vi "PCO_SetConfig.vi"(8 "error in":errorcluster caption="entrée d'erreur", 11 "PCO_Config":T3 {"TriggerMode" items=["auto sequence", "software trigger", "external exposure start", "external exposure control"]}) -> (0 "error out":errorcluster caption="sortie d'erreur", 1 "PCO_Config 2":T3 {"TriggerMode" items=["auto sequence", "software trigger", "external exposure start", "external exposure control"]}, 2 "Trigger externe?":bool, 3 "configuration":T2={"exposure_time_s"=nan, "delay_time_s"=nan, "roi"={"x0"=18446744073709551615, "y0"=18446744073709551615, "x1"=18446744073709551615, "y1"=18446744073709551615}, "timestamp_mode"=65535, "pixelrate"=4294967295, "conversion_factor"=0.7, "trigger_mode"=65535, "acquire_mode"=65535, "acquire_sequence_number"=1, "metadata_mode"=65535, "noisefilter_mode"=65535, "pixel_format"=0, "binning"={"vert"=0, "horz"=0, "mode"=0}, "auto_exposure"={"region"=0, "min_exposure_s"=0.001, "max_exposure_s"=0.1}} {"conversion_factor" format="%.2g"; "auto_exposure"."region" items=["balanced", "center_based", "corner_based", "full", "custom"]; "binning"."mode" items=["sum", "average"]; "noisefilter_mode" items=["Undefined"=65535, "OFF"=0, "ON"=1]; "exposure_time_s" format="%#_6f"; "timestamp_mode" items=["Undefined"=65535, "OFF"=0, "Binary"=1, "Binary+ASCII"=2, "ASCII"=3]; "acquire_mode" items=["Undefined"=65535, "auto"=0, "external"=1, "external modulate"=2]; "trigger_mode" items=["Undefined"=65535, "auto sequence"=0, "software trigger"=1, "external exposure start & software trigger"=2, "external exposure control"=3, "external synchronized"=4, "fast external exposure control"=5, "external CDS control"=6, "slow external exposure control"=7, "external synchronized HDSDI"=258]; "metadata_mode" items=["Undefined"=65535, "OFF"=0, "ON"=1]})   [LabVIEW 2026]
uses:
  Controls/PCO_Config.ctl
  pco.labview/camera/Controls/binning.ctl
  pco.labview/camera/Camera.lvclass
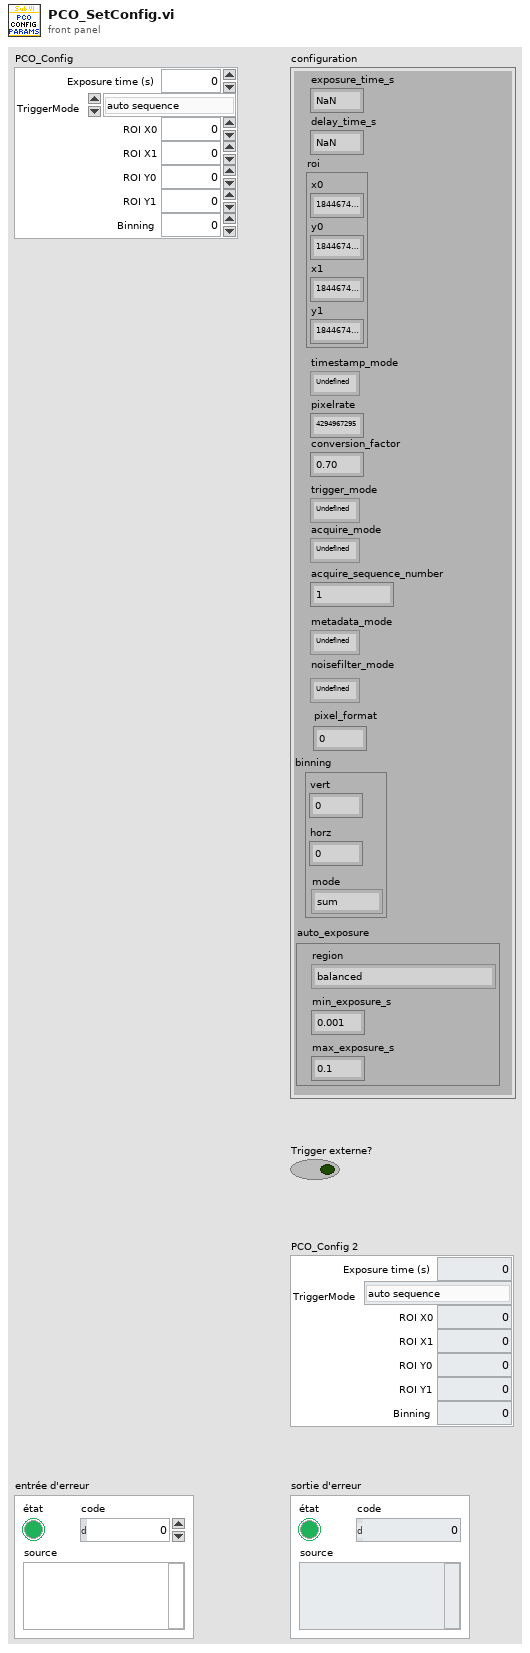
[diagram p1: front panel]
types:
  T1 = typedef "Camera.lvclass/binning.ctl" = cluster{"vert":u16, "horz":u16, "mode":u16}
  T2 = cluster{"exposure_time_s":dbl, "delay_time_s":dbl, "roi":cluster{"x0":u64, "y0":u64, "x1":u64, "y1":u64}, "timestamp_mode":u16, "pixelrate":u32, "conversion_factor":sgl, "trigger_mode":u16, "acquire_mode":u16, "acquire_sequence_number":u32, "metadata_mode":u16, "noisefilter_mode":u16, "pixel_format":u32, "binning":T1, "auto_exposure":cluster{"region":u16, "min_exposure_s":dbl, "max_exposure_s":dbl}}
  T3 = typedef "PCO_Config.ctl" = cluster{"Exposure time (s)":dbl, "TriggerMode":u16, "ROI X0":u16, "ROI Y0":u16, "ROI X1":u16, "ROI Y1":u16, "Binning":u8}
  T4 = enum16{"auto sequence", "software trigger", "external exposure start", "external exposure control"}
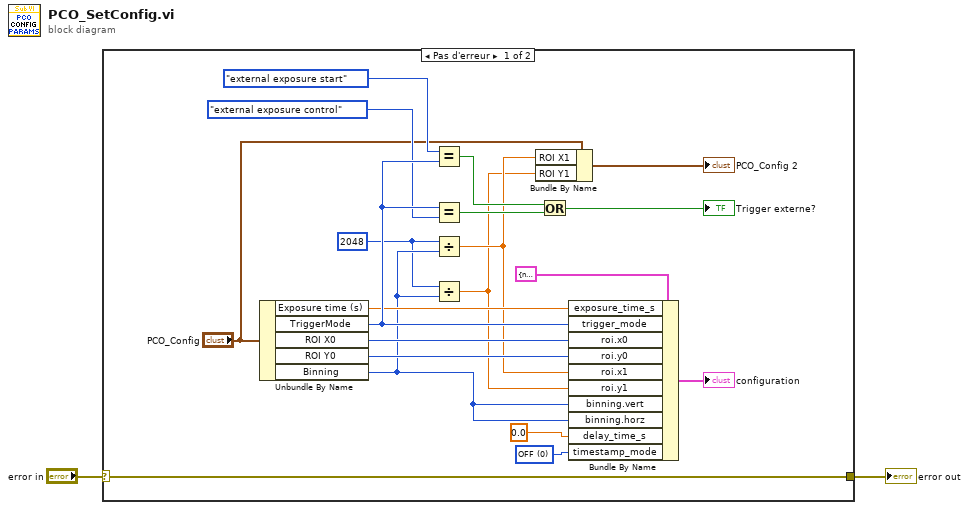
[diagram p0: block diagram]
diagram:
  n1 = case shown="Pas d'erreur" "error in" {
    selector: "error in" -> [w11 w23]
    tunnel: [w11 w23] -> w1
    frame No Error {
      w9 = 2048
      w14 = u16 0 items=["OFF", "Binary", "Binary+ASCII", "ASCII"] ("wTimeStampMode")
      n2 = Unbundle By Name("PCO_Config") -> ("Exposure time (s)"=w12:dbl, "TriggerMode"=w21:u16, "ROI X0"=w15:u16, "ROI Y0"=w16:u16, "Binning"=w10:u8)
      n3 = Equal?(x=T4."external exposure start" ("TriggerMode"), y=w21) -> (x = y?=w19:bool)
      n4 = Equal?(x=w21, y=T4."external exposure control" ("TriggerMode")) -> (x = y?=w20:bool)
      n5 = Divide(x=w9, y=w10) -> (x/y=w6:dbl)
      n6 = Divide(x=w9, y=w10) -> (x/y=w5:dbl)
      n7 = Bundle By Name(cluster="PCO_Config", "ROI X1"=w6, "ROI Y1"=w5) -> (→"PCO_Config 2":T3)
      n8 = Or(x=w19, y=w20) -> (x .or. y?=→"Trigger externe?":bool)
      n9 = Bundle By Name(cluster=T2 {"exposure_time_s"=nan, "delay_time_s"=nan, "roi"={"x0"=18446744073709551615, "y0"=18446744073709551615, "x1"=18446744073709551615, "y1"=18446744073709551615}, "timestamp_mode"=65535, "pixelrate"=4294967295, "conversion_factor"=0.7, "trigger_mode"=65535, "acquire_mode"=65535, "acquire_sequence_number"=1, "metadata_mode"=65535, "noisefilter_mode"=65535, "pixel_format"=0, "binning"={"vert"=0, "horz"=0, "mode"=0}, "auto_exposure"={"region"=0, "min_exposure_s"=0.001, "max_exposure_s"=0.1}} ("configuration 2"), "exposure_time_s"=w12, "trigger_mode"=w21, "roi.x0"=w15, "roi.y0"=w16, "roi.x1"=w6, "roi.y1"=w5, "binning.vert"=w10, "binning.horz"=w10, "delay_time_s"=0.0, "timestamp_mode"=w14) -> (→"configuration":T2)
    }
    frame Error {
    }
  }
  "error out" <- w1
